vi "Make_Saw_Invert.vi"(1 "N_steps_1":i32 min=0 step=1) -> (0 "SawInvertWaveform":dbl[](array[numeric]))   [LabVIEW 2019]
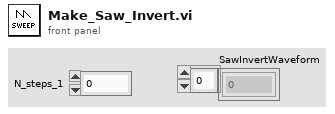
[diagram p1: front panel]
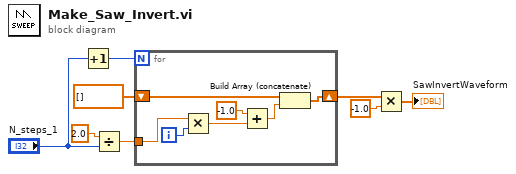
[diagram p0: block diagram]
diagram:
  n1 = Increment(x="N_steps_1") -> (x+1=w5:i32)
  n2 = Divide(x=2.0, y="N_steps_1") -> (x/y=w7:dbl)
  n3 = for {
    N: w5 -> [_]
    tunnel: w7 -> [w13]
    shift-right: [w10] -> w2
    shift-left: dbl[] [] -> [w11]
    i -> [w14]
    n4 = Multiply(x=w13, y=w14) -> (x*y=w12:dbl)
    n5 = Add(x=-1.0, y=w12) -> (x+y=w9:dbl)
    n6 = Build Array (concatenate)(w11, w9) -> (w10:dbl[])
  }
  n7 = Multiply(x=w2, y=-1.0) -> (x*y=→"SawInvertWaveform":dbl[])
